vi "Get Number of Arrangements.vi"(8 "error in (no error)":errorcluster, 10 "Group Sizes":i64[](array[numeric]), 11 "Proto in":refnum<class "Group.lvclass">) -> (0 "error out":errorcluster, 2 "Arrangements":u64, 3 "Proto out":refnum<class "Group.lvclass">)   [LabVIEW 2021, in "Group.lvclass"]
uses:
  Group.lvclass
  Group.lvclass/Group.ctl
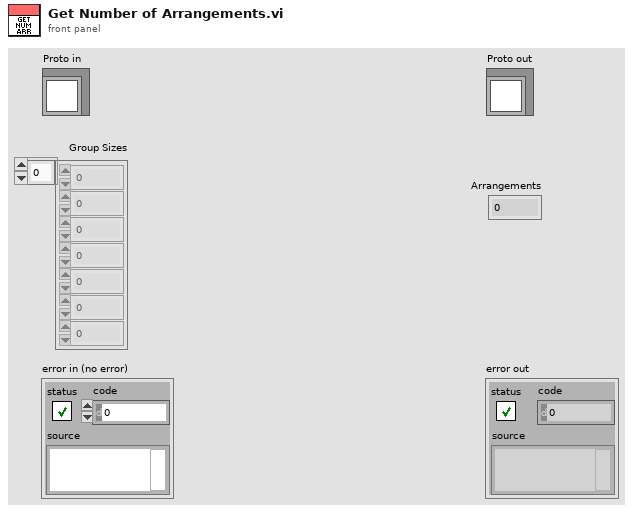
[diagram p1: front panel]
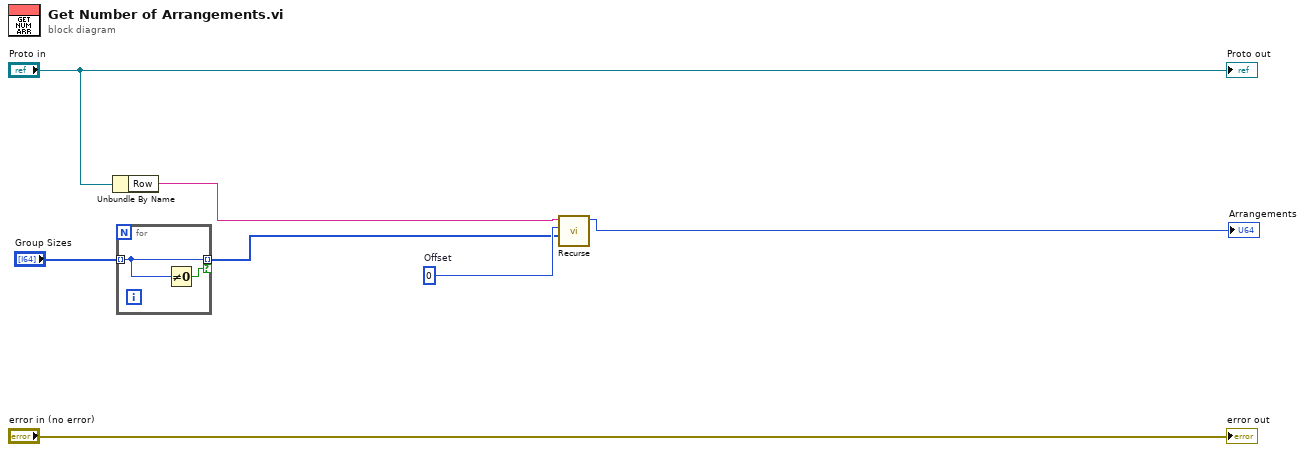
[diagram p0: block diagram]
diagram:
  w3 = 0  # Offset
  n1 = Unbundle By Name("Proto in") -> ("Row"=w5:string)
  n2 = for {
    tunnel: "Group Sizes" -> [w9] mode=indexing
    tunnel: [w9] -> w1 mode=indexing if=w8
    n3 = Not Equal To 0?(x=w9) -> (x != 0?=w8:bool)
  }
  n4 = call "Recurse.vi"("Group Sizes"=w1, "Offset"=w3, "Row"=w5) -> ("Number of aranagements"=→"Arrangements":u64)  [unwired: 8 in]
  "error out" <- "error in (no error)"
  "Proto out" <- "Proto in"
